vi "SecondMarkerRole.vi"(7 "firstCall":bool, 10 "Game in":refnum<class "Game.lvclass">, 11 "SecondMarkerRole":refnum<class "SecondMarkerRole.lvclass">) -> (1 "Game out":refnum<class "Game.lvclass">, 2 "Robot out":refnum<class "Robot.lvclass">, 3 "SecondMarkerRole 2":refnum<class "SecondMarkerRole.lvclass">)   [LabVIEW 2023, in "SecondMarkerRole.lvclass"]
uses:
  SecondMarkerRole.lvclass
  Game_class/Game.lvclass
  Robot_class/Robot.lvclass
  C:/Users/ebert/Desktop/roboime/SSL_AI/Role_class/Role.lvclass
  Role_class/Role.lvclass/Role.ctl
  MarkerTactic_class/MarkerTacticStates.ctl
  Tacticbook_class/Tacticbook.lvclass/Tacticbook.ctl
  Tacticbook_class/Read MarkerTactic.vi
  Tacticbook_class/Write MarkerTactic.vi
  Role_class/Read Tacticbook.vi
  Role_class/Write Tacticbook.vi
  Role_class/Write tactic_index.vi
  Role_class/Read RobotRef.vi
  Tacticbook_class/Tacticbook.lvclass
  MarkerTactic_class/MarkerTactic.lvclass
panel:
  out "error out":errorcluster
  in  "error in (no error)":errorcluster
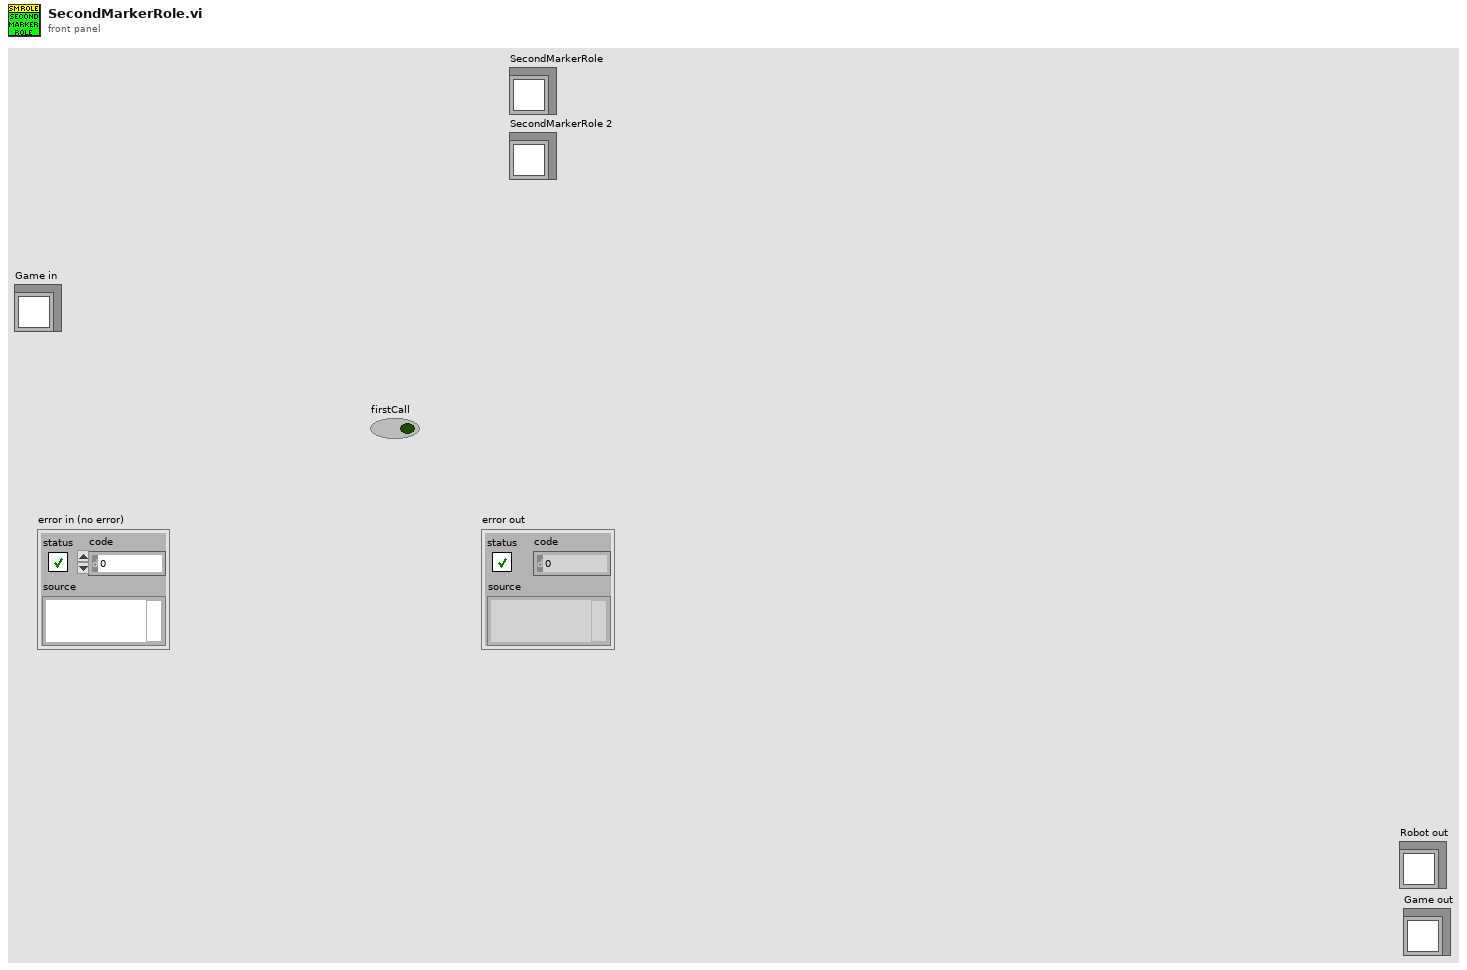
[diagram p1: front panel]
types:
  T1 = typedef "MarkerTacticStates.ctl" = enum16{"Exit", "BlockOurGoal", "FollowAttacker", "BlockEnemyPass"}
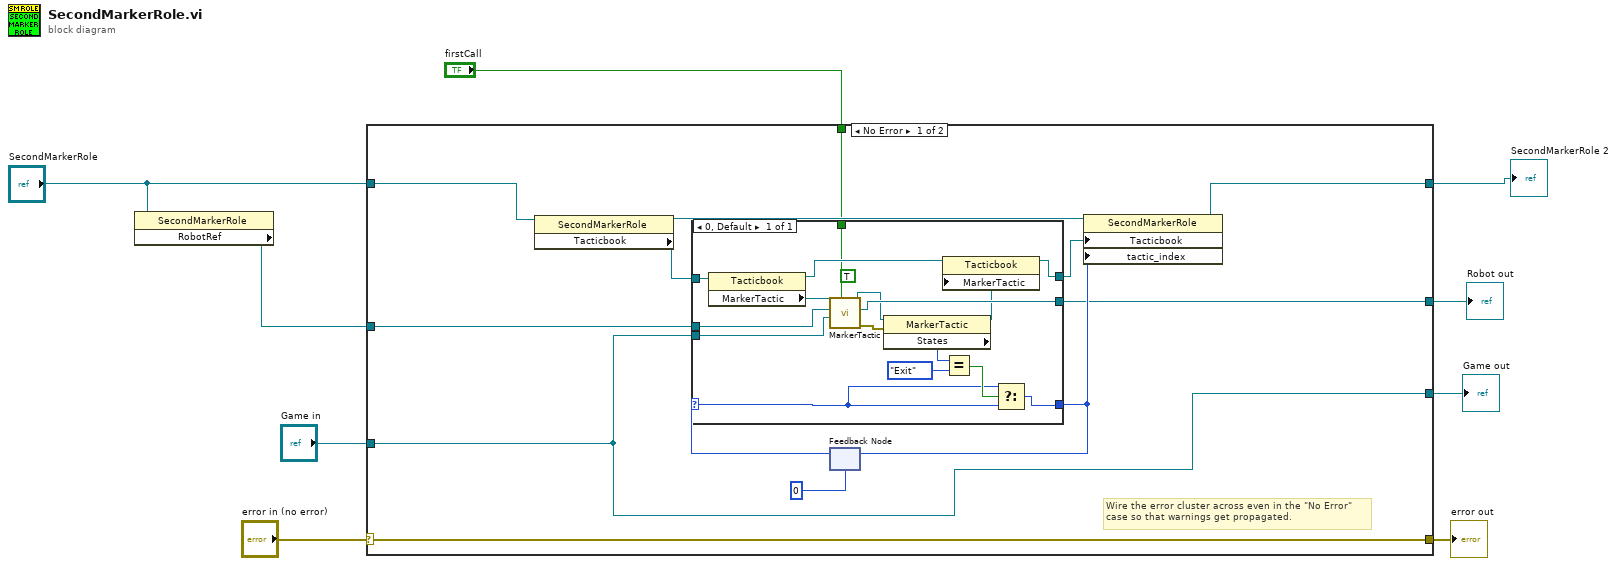
[diagram p0: block diagram]
diagram:
  n1 = property class="SecondMarkerRole"(reference="SecondMarkerRole") -> ("RobotRef"=w4:refnum<class "Robot.lvclass">)  [unwired: 1 in, 2 out]
  n2 = case shown="No Error" "error in (no error)" {
    selector: "error in (no error)" -> [w22 w41]
    tunnel: [w22 w41] -> w8
    tunnel: [w14 w40] -> w1
    tunnel: "SecondMarkerRole" -> [w15 w40]
    tunnel: "Game in" -> [w12 w39]
    tunnel: [w13 _] -> w6
    tunnel: [w12 w39] -> w5
    tunnel: w4 -> [w11 _]
    tunnel: "firstCall" -> [w10 _]
    frame No Error {
      # "Wire the error cluster across even in the \"No Error\"\ncase so that warnings get propagated."
      n3 = property class="SecondMarkerRole"(reference=w15) -> (reference out=w21:refnum<class "SecondMarkerRole.lvclass">, "Tacticbook"=w18:refnum<class "Tacticbook.lvclass">)  [unwired: 1 in, 1 out]
      n4 = feedback #1(0) -> (w19:i32)
      n5 = case shown="0, Default" w19 {
        selector: w19 -> [w25]
        tunnel: [w31] -> w17
        tunnel: w18 -> [w38]
        tunnel: [w36] -> w13
        tunnel: [w28] -> w16
        tunnel: w12 -> [w27]
        tunnel: w11 -> [w26]
        tunnel: w10 -> [w23]
        frame 0, Default {
          (unwired) TRUE ("SecondMostDangerous")
          n6 = property class="Tacticbook"(reference=w38) -> (reference out=w30:refnum<class "Tacticbook.lvclass">, "MarkerTactic"=w37:refnum<class "MarkerTactic.lvclass">)  [unwired: 1 in, 1 out]
          n7 = call "MarkerTactic.vi"("firstCall"=w23, "Game in"=w27, "Robot"=w26, "MarkerTactic in"=w37) -> ("error out"=w35:errorcluster, "Robot out"=w36:refnum<class "Robot.lvclass">, "MarkerTactic out"=w34:refnum<class "MarkerTactic.lvclass">)  [unwired: 5 in]
          n8 = property class="MarkerTactic"(reference=w34, error in=w35) -> (reference out=w29:refnum<class "MarkerTactic.lvclass">, "States"=w33:T1)  [unwired: 1 out]
          n9 = property class="Tacticbook"(reference=w30, "MarkerTactic"=w29) -> (reference out=w28:refnum<class "Tacticbook.lvclass">)  [unwired: 1 in, 1 out]
          n10 = Equal?(x=w33, y=MarkerTacticStates."Exit") -> (x = y?=w32:bool)
          n11 = Select(t=w25, s=w32, f=w25) -> (s? t:f=w31:i32)
        }
      }
      n12 = feedback-in #1(w17) -> ()
      n13 = property class="SecondMarkerRole"(reference=w21, "Tacticbook"=w16, "tactic_index"=w17) -> (reference out=w14:refnum<class "SecondMarkerRole.lvclass">)  [unwired: 1 in, 1 out]
    }
    frame Error {
    }
  }
  "error out" <- w8
  "Robot out" <- w6
  "Game out" <- w5
  "SecondMarkerRole 2" <- w1
